vi "Tree to Variant.vi"(10 "Name":string="untitled", 11 "Variant Tree":variant) -> (3 "Variant":variant)   [LabVIEW 2013, in "OpenVariant.lvlib"]
uses:
  TypeDescriptor/TypeDescriptor_GetName.vi
  TypeDescriptor/TypeDescriptor_GetType.vi
  TypeDescriptor/TypeDescriptor_GetPString.vi
  <vilib>/Utility/VariantDataType/GetTypeInfo.vi
  <vilib>/Utility/GetType.llb/TD_Create Cluster.vi
  TypeDescriptor/TypeDescriptor_SetName.vi
  OpenVariant.lvlib
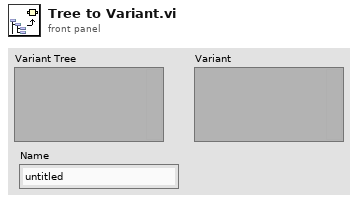
[diagram p1: front panel]
types:
  T1 = typedef "VariantType.lvlib/Type.ctl" = enum8{"Invalid Type", "Void", "I8", "I16", "I32", "I64", "U8", "U16", "U32", "U64", "Single Float", "Double Float", "Extended Float", "Single Complex", "Double Complex", "Extended Complex", "Enum U8", "Enum U16", "Enum U32", "Enum U64", "Single Float With Unit", "Double Float With Unit", "Extended Float With Unit", "Single Complex with Unit", "Double Complex with Unit", "Extended Complex with Unit", "Boolean", "String", "Path", "Picture", "Tag", "Array", "Cluster", "Variant", "LV Variant", "Waveform", "Timestamp", "Digital Waveform", "Digital Data", "ExpressData", "Refnum", "External Data", "VI", "Poly VI", "LabVIEW Class Instance", "Fixed Point"}
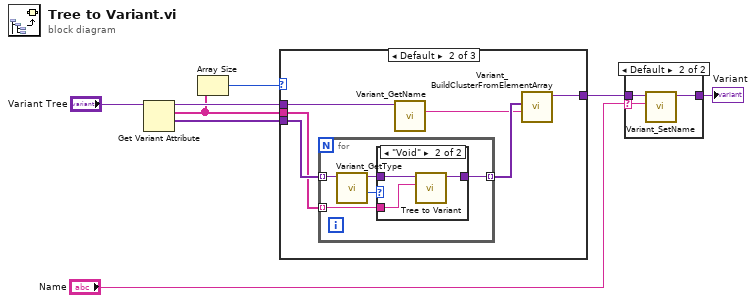
[diagram p0: block diagram]
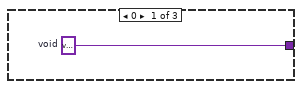
[diagram p3: hidden frame]
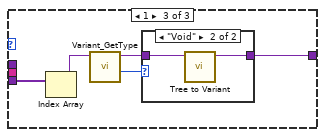
[diagram p5: hidden frame]
diagram:
  n1 = Get Variant Attribute(Variant="Variant Tree") -> (duplicate Variant=w8:variant, names=w5:string[], values=w4:variant[])  [unwired: 3 in, 1 out]
  n2 = Array Size(array=w5) -> (size(s)=w6:i32)
  n3 = case shown="Default" w6 {
    tunnel: w4 -> [_ w15 w29]
    tunnel: w5 -> [_ w10 _]
    tunnel: [w9 w11 w26] -> w2
    tunnel: w8 -> [_ w14 _]
    frame 0 {
      w9 = variant  # void
    }
    frame Default {
      n4 = for {
        tunnel: w15 -> [w20] mode=indexing
        tunnel: [w17] -> w13 mode=indexing
        tunnel: w10 -> [w16] mode=indexing
        n5 = call "Variant_GetType.vi"("Variant"=w20) -> ("LV Type Enum"=w18:T1, "Variant dup"=w19:variant)  [unwired: 8 in, 1 out]
        n6 = case shown="\"Void\"" w18 {
          tunnel: w19 -> [w21 w24]
          tunnel: [w21 w23] -> w17
          tunnel: w16 -> [_ w22]
          frame Default {
          }
          frame "Void" {
            n7 = call "Tree to Variant.vi"("Name"=w22, "Variant Tree"=w24) -> ("Variant"=w23:variant)  [unwired: 9 in]
          }
        }
      }
      n8 = call "Variant_GetName.vi"("Variant"=w14) -> ("Name"=w12:string)  [unwired: 8 in, 2 out]
      n9 = call "Variant_BuildClusterFromElementArray.vi"("name"=w12, "Elements"=w13) -> ("Cluster"=w11:variant)  [unwired: 9 in]
    }
    frame 1 {
      n10 = Index Array(array=w29) -> (element=w25:variant)  [unwired: 1 in]
      n11 = call "Variant_GetType.vi"("Variant"=w25) -> ("LV Type Enum"=w27:T1, "Variant dup"=w28:variant)  [unwired: 8 in, 1 out]
      n12 = case shown="\"Void\"" w27 {
        tunnel: w28 -> [w30 w32]
        tunnel: [w30 w31] -> w26
        frame Default {
        }
        frame "Void" {
          n13 = call "Tree to Variant.vi"("Variant Tree"=w32) -> ("Variant"=w31:variant)  [unwired: 10 in]
        }
      }
    }
  }
  n14 = case shown="Default" "Name" {
    selector: "Name" -> [_ w34]
    tunnel: [w33 w36] -> w3
    tunnel: w2 -> [w33 w35]
    frame "\u0000" {
    }
    frame Default {
      n15 = call "Variant_SetName.vi"("Name"=w34, "Variant"=w35) -> ("Named Variant"=w36:variant)  [unwired: 9 in]
    }
  }
  "Variant" <- w3
